vi "SET CONFIGURATIO.vi"(8 "error in (no error)":errorcluster, 9 "MONEY":cluster{"COIN":string, "VALUE":dbl}, 10 "PRODUCTS":T1, 11 "MONEY ARRAY":string[](array[string])) -> (0 "error out":errorcluster, 1 "MONEY OUT":cluster{"COIN":string, "VALUE":dbl}, 2 "PRODUCTS OUT":T1, 3 "MONEY ARRAY OUT":string[](array[string]))   [LabVIEW 2019, in "CONFIGURATION.lvlib"]
doc: "HERE WE CAN SET OUR PRODUCT AND MONEY CONFIGURATION\n_____\nCreated using Delacor QMH Event Scripter 5.0.0.112."
uses:
  CONFIGURATION.lvlib
  SET CONFIGURATIO Argument--cluster.ctl
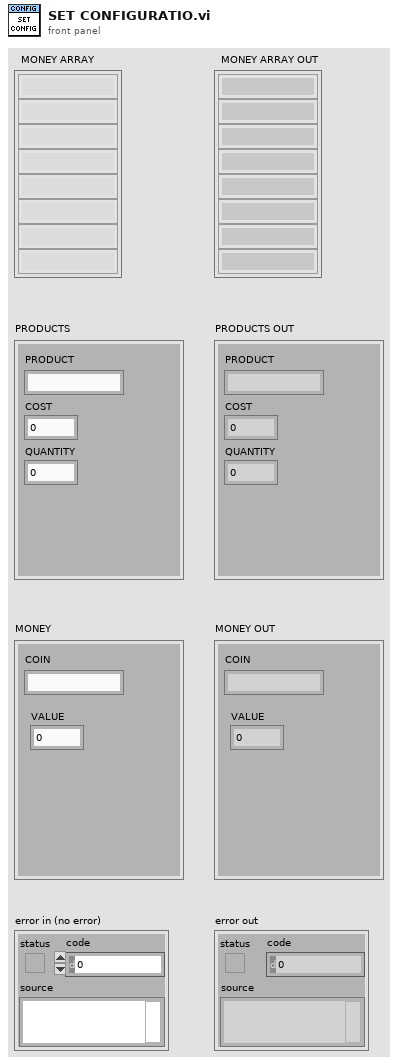
[diagram p1: front panel]
types:
  T1 = cluster{"PRODUCT":string, "COST":dbl, "QUANTITY":i8}
  T2 = typedef "CONFIGURATION.lvlib/SET CONFIGURATIO Argument--cluster.ctl" = cluster{"PRODUCTS":cluster{"PRODUCT":string, "COST":dbl, "QUANTITY":i8}, "MONEY":cluster{"COIN":string, "VALUE":dbl}, "MONEY ARRAY":string[]}
  T3 = typedef "CONFIGURATION.lvlib/Request Events--cluster.ctl" = cluster{"Stop Module":refnum<user-event>, "Show Panel":refnum<user-event>, "Hide Panel":refnum<user-event>, "Get Module Execution Status":refnum<user-event>, "Show Diagram":refnum<user-event>, "SET CONFIGURATIO":refnum<user-event>, "UPDATE DB TO MONEY LIST":refnum<user-event>, "SAVE IN DB":refnum<user-event>, "SAVE PRODUCT IN DATABASE":refnum<user-event>, "UPDATE DB TO PRODUCT LIST":refnum<user-event>}
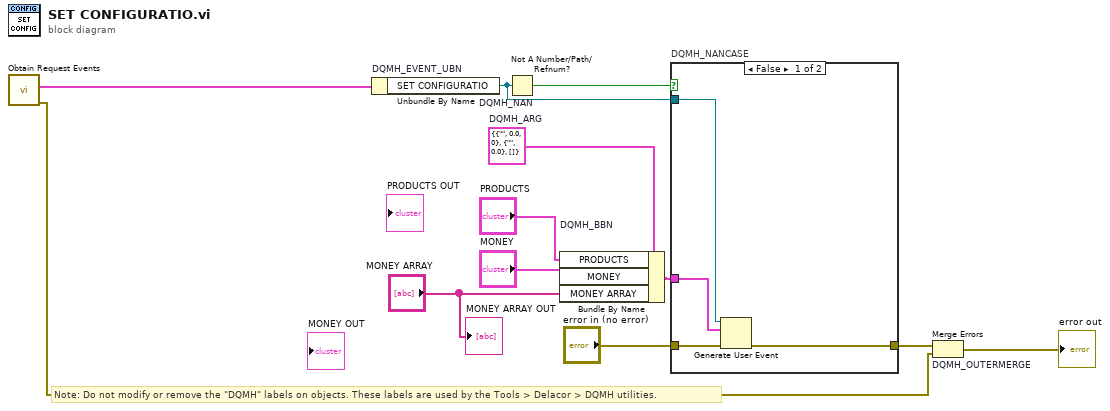
[diagram p0: block diagram]
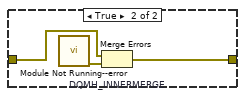
[diagram p2: hidden frame]
diagram:
  w6 = T2 {"PRODUCTS"={"PRODUCT"="", "COST"=0.0, "QUANTITY"=0}, "MONEY"={"COIN"="", "VALUE"=0.0}, "MONEY ARRAY"=[]}  # DQMH_ARG
  # "Note: Do not modify or remove the \"DQMH\" labels on objects. These labels are used by the Tools > Delacor > DQMH utilities."
  n1 = call "Obtain Request Events.vi"() -> ("error out"=w3:errorcluster, "CONFIGURATION Request Events"=w2:T3)  [unwired: 10 in]
  n2 = Unbundle By Name "DQMH_EVENT_UBN"(w2) -> ("SET CONFIGURATIO"=w8:refnum<user-event>)
  n3 = Not A Number/Path/Refnum? "DQMH_NAN"(number/path/refnum=w8) -> (NaN/Path/Refnum?=w9:bool)
  n4 = Bundle By Name "DQMH_BBN"(cluster=w6, "PRODUCTS"="PRODUCTS", "MONEY"="MONEY", "MONEY ARRAY"="MONEY ARRAY") -> (w10:T2)
  n5 = case "DQMH_NANCASE" shown="False" w9 {
    tunnel: "error in (no error)" -> [w16 w19]
    tunnel: [w15 w18] -> w7
    tunnel: w8 -> [w14 _]
    tunnel: w10 -> [w13 _]
    frame False {
      n6 = Generate User Event(user event=w14, event data cluster=w13, error in=w16) -> (error out=w15:errorcluster)  [unwired: 1 in, 1 out]
    }
    frame True {
      n7 = call "Module Not Running--error.vi"() -> ("error out"=w17:errorcluster)  [unwired: 11 in]
      n8 = Merge Errors "DQMH_INNERMERGE"(w19, w17) -> (w18:errorcluster)
    }
  }
  n9 = Merge Errors "DQMH_OUTERMERGE"(w7, w3) -> (→"error out":errorcluster)
  "MONEY ARRAY OUT" <- "MONEY ARRAY"
